vi "Begin.vi"() -> (0 "error out":errorcluster)   [LabVIEW 2013]
doc: "Called before other user functions, this VI is expected to open initial I/O refnums, load in file data, and do all program initialization. Notice that the <B>error out</B> terminal is simply used for data flow. Wiring it to other structures or subVIs ensures that this VI runs first."
uses:
  <vilib>/Rock Robotics/WPI/Joystick/WPI_JoystickDeviceEnum.ctl
  <vilib>/Rock Robotics/SystemInterfaces/Typedef/FPGA_TypedefDigitalModule.ctl
  <vilib>/Rock Robotics/SystemInterfaces/DIO/FPGA_DIOChannel.ctl
  <vilib>/Rock Robotics/SystemInterfaces/DIO/FPGA_DIORelayChannel.ctl
  <vilib>/Rock Robotics/SystemInterfaces/Typedef/FPGA_TypedefSolenoidModule.ctl
  <vilib>/Rock Robotics/WPI/Solenoid/WPI_SolenoidChannel.ctl
  <vilib>/Rock Robotics/WPI/Solenoid/WPI_SolenoidValue.ctl
  <vilib>/Rock Robotics/SystemInterfaces/DIO/FPGA_DIOPWMChannel.ctl
  <vilib>/Rock Robotics/WPI/Solenoid/WPI_SolenoidOpenDouble.vi
  <vilib>/Rock Robotics/WPI/Solenoid/WPI_SolenoidSetEnum.vi
  <vilib>/Rock Robotics/WPI/Counter/WPI_CounterDigitalInputToDigitalSource.vi
  <vilib>/Rock Robotics/WPI/RobotDrive/WPI_RobotDriveOpen2MotorWithVictor.vi
  <vilib>/Rock Robotics/WPI/Compressor/WPI_CompressorGetSetRefNum.vi
  <vilib>/Rock Robotics/WPI/Camera/WPI_CameraImageSize.ctl
  <vilib>/Rock Robotics/WPI/Camera/WPI_CameraWhite Balance Values.ctl
  <vilib>/Rock Robotics/WPI/Camera/WPI_CameraExposure Values.ctl
  <vilib>/Rock Robotics/WPI/Camera/WPI_CameraFrameRate.ctl
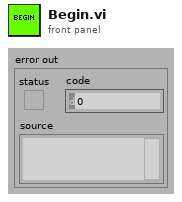
[diagram p1: front panel]
types:
  T1 = typedef "FPGA_DIOChannel.ctl" = enum8{"DIO 1", "DIO 2", "DIO 3", "DIO 4", "DIO 5", "DIO 6", "DIO 7", "DIO 8", "DIO 9", "DIO 10", "DIO 11", "DIO 12", "DIO 13", "DIO 14", "Invalid"}
  T2 = typedef "FPGA_DIOPWMChannel.ctl" = enum8{"PWM 1", "PWM 2", "PWM 3", "PWM 4", "PWM 5", "PWM 6", "PWM 7", "PWM 8", "PWM 9", "PWM 10", "Invalid"}
  T3 = typedef "WPI_SolenoidValue.ctl" = enum16{"Off", "On", "Forward", "Reverse"}
  T4 = typedef "WPI_SolenoidChannel.ctl" = enum8{"Solenoid 1", "Solenoid 2", "Solenoid 3", "Solenoid 4", "Solenoid 5", "Solenoid 6", "Solenoid 7", "Solenoid 8", "Invalid"}
  T5 = typedef "FPGA_TypedefSolenoidModule.ctl" = enum16{"Solenoid Module 1", "Solenoid Module 2"}
  T6 = typedef "FPGA_DIORelayChannel.ctl" = enum8{"Relay 1", "Relay 2", "Relay 3", "Relay 4", "Relay 5", "Relay 6", "Relay 7", "Relay 8", "Invalid"}
  T7 = typedef "WPI_JoystickDeviceEnum.ctl" = enum16{"USB 1", "USB 2", "USB 3", "USB 4", "Kinect 1", "Kinect 2"}
  T8 = typedef "FPGA_TypedefDigitalModule.ctl" = enum16{"Digital Module 1", "Digital Module 2"}
  T9 = typedef "WPI_CameraFrameRate.ctl" = u32
  T10 = typedef "WPI_CameraExposure Values.ctl" = enum16{"Auto", "Flicker-free 50 Hz", "Flicker-free 60 Hz", "Hold current"}
  T11 = typedef "WPI_CameraWhite Balance Values.ctl" = enum16{"Auto", "Fixed indoor", "Fixed outdoor 1", "Fixed outdoor 2", "Fixed fluorescent 1", "Fixed fluorescent 2", "Hold current"}
  T12 = typedef "WPI_CameraImageSize.ctl" = enum16{"640x480", "320x240", "160x120"}
  T13 = typedef "WPI_CameraDevRef.ctl" = cluster{"Camera Address":string, "CameraStatus":errorcluster, "Acquire Image Notifier":refnum<notifier>}
  T14 = typedef "WPI_SolenoidDevRef.ctl" = cluster{"DevStatus":errorcluster, "Solenoid Module":T5, "Forward Solenoid Channel":T4, "Reverse Solenoid Channel":T4}
  T15 = typedef "WPI_DigitalInputDevRef.ctl" = cluster{"DevStatus":errorcluster, "DIO Channel":T1, "Digital Module":T8}
  T16 = typedef "WPI_RobotDriveDevRef.ctl" = cluster{"DevStatus":errorcluster, "Motors[]":T17[], "Square Inputs":bool, "Max Output":dbl, "Isochronous":bool}
  T17 = typedef "WPI_MotorControlDeviceRef.ctl" = cluster{"DeviceStatus":errorcluster, "Type":enum16{"PWM", "CAN"}, "PWM":cluster{"Digital Module":T8, "PWM Channel":T2, "DeadBand":T18}, "CAN":cluster{"Device Number":u8, "Control Mode":T19, "Semaphore":T20, "Max Vout":dbl}, "Invert":bool, "TransformRef":T21, "InvTransformRef":T21}
  T18 = typedef "WPI_PWMDeadband.ctl" = cluster{"Name":string, "maxPositivePwm":i32, "minPositivePwm":i32, "centerPwm":i32, "maxNegativePwm":i32, "minNegativePwm":i32, "angularRange":u16}
  T19 = typedef "WPI_CANJaguar_ControlMode.ctl" = enum8{"Percent VBus", "Current", "Speed", "Position", "Voltage"}
  T20 = typedef "Semaphore RefNum" = refnum<k1>
  T21 = typedef "WPI_PWMTransform_ConPane.ctl" = refnum<vi>
  T22 = typedef "WPI_CompressorDevRef.ctl" = cluster{"DevStatus":errorcluster, "DigitalInputDevRef":T15, "RelayDevRef":T23}
  T23 = typedef "WPI_RelayDevRef.ctl" = cluster{"DevStatus":errorcluster, "Relay Channel":T6, "Digital Module":T8, "Relay Direction":T24}
  T24 = typedef "WPI_RelayDirection.ctl" = enum16{"Both directions", "Forward only", "Reverse only"}
  T25 = typedef "FPGA_CounterEncoderSourceConvertionLVSourceType.ctl" = cluster{"DevStatus":errorcluster, "AnalogTriggerMode?":bool, "DigitalMode":cluster{"Digital Module":T8, "DIO Channel":T26}, "AnalogTriggerMode":cluster{"AnalogTriggerIndex":T27, "OutputType":T28}}
  T26 = typedef "FPGA_DIODigitalSourceChannel.ctl" = enum8{"DIO 1", "DIO 2", "DIO 3", "DIO 4", "DIO 5", "DIO 6", "DIO 7", "DIO 8", "DIO 9", "DIO 10", "DIO 11", "DIO 12", "DIO 13", "DIO 14", "Disabled"}
  T27 = typedef "FPGA_AnalogTriggerIndex.ctl" = enum8{"Trig 0", "Trig 1", "Trig 2", "Trig 3", "Trig 4", "Trig 5", "Trig 6", "Trig 7", "Invalid"}
  T28 = typedef "FPGA_AnalogTriggerOutType.ctl" = enum16{"InWindow", "TriggerState", "Rising", "Falling"}
  T29 = typedef "WPI_EncoderDevRef.ctl" = cluster{"DevStatus":errorcluster, "EncoderIndex":T30, "CounterIndex":T31, "DistancePerCount":dbl, "Decoding Type":T32}
  T30 = typedef "FPGA_EncoderIdx.ctl" = enum8{"Enc 0", "Enc 1", "Enc 2", "Enc 3", "Invalid"}
  T31 = typedef "FPGA_CounterCtrSystemIndex.ctl" = enum8{"Ctr 0", "Ctr 1", "Ctr 2", "Ctr 3", "Ctr 4", "Ctr 5", "Ctr 6", "Ctr 7", "Invalid"}
  T32 = typedef "WPI_EncoderType.ctl" = enum16{"1x", "2x", "4x"}
  T33 = typedef "WPI_JoystickDevRef.ctl" = cluster{"Device":T7}
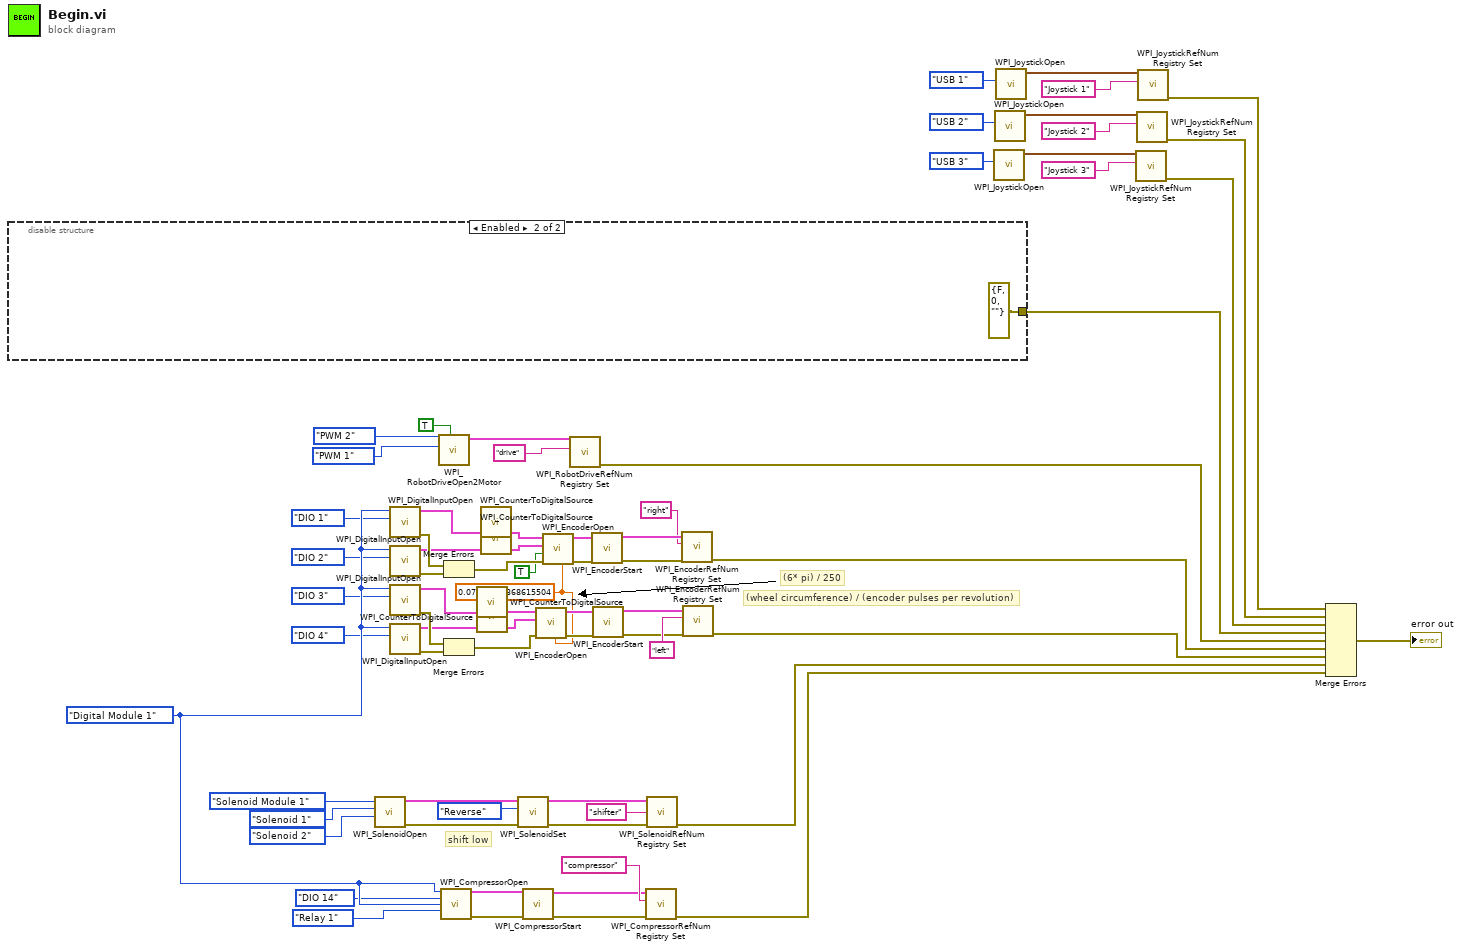
[diagram p0: block diagram]
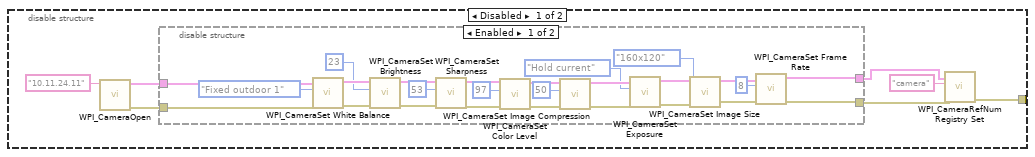
[diagram p2: hidden frame]
diagram:
  w11 = 0.07539822368615504 ("DistancePerCount")
  w54 = FPGA_TypedefDigitalModule."Digital Module 1" ("Digital Module (Module 1)")
  # "shift low"
  # "(wheel circumference) / (encoder pulses per revolution)"
  # "(6* pi) / 250"
  n1 = disable-structure shown="Enabled" {
    disable-tunnel: [w72 errorcluster {"status"=FALSE, "code"=0, "source"=""} ("error out")] -> w59
    frame Disabled {
      n2 = call <vilib>:"WPI_CameraOpen.vi"("Camera Address"="10.11.24.11") -> ("error out"=w74:errorcluster, "CameraDevRef"=w76:T13)  [unwired: 9 in]
      n3 = disable-structure shown="Enabled" {
        disable-tunnel: w76 -> [w102 w106]
        disable-tunnel: [w80 w106] -> w75
        disable-tunnel: w74 -> [w89 w105]
        disable-tunnel: [w79 w105] -> w73
        frame Enabled {
          n4 = call <vilib>:"WPI_CameraSet White Balance.vi"("error in (no error)"=w89, "White Balance"=WPI_CameraWhite_Balance_Values."Fixed outdoor 1", "CameraDevRef"=w102) -> ("error out"=w90:errorcluster, "CameraDevRef Out"=w101:T13)  [unwired: 7 in]
          n5 = call <vilib>:"WPI_CameraSet Brightness.vi"("error in (no error)"=w90, "Brightness"=23, "CameraDevRef"=w101) -> ("error out"=w91:errorcluster, "CameraDevRef Out"=w100:T13)  [unwired: 7 in]
          n6 = call <vilib>:"WPI_CameraSet Sharpness.vi"("error in (no error)"=w91, "Sharpness"=53, "CameraDevRef"=w100) -> ("error out"=w92:errorcluster, "CameraDevRef Out"=w99:T13)  [unwired: 7 in]
          n7 = call <vilib>:"WPI_CameraSet Color Level.vi"("error in (no error)"=w92, "Color Level"=97, "CameraDevRef"=w99) -> ("error out"=w93:errorcluster, "CameraDevRef Out"=w98:T13)  [unwired: 7 in]
          n8 = call <vilib>:"WPI_CameraSet Image Compression.vi"("error in (no error)"=w93, "Compression"=50, "CameraDevRef"=w98) -> ("error out"=w104:errorcluster, "CameraDevRef Out"=w103:T13)  [unwired: 7 in]
          n9 = call <vilib>:"WPI_CameraSet Exposure.vi"("error in (no error)"=w104, "Exposure"=WPI_CameraExposure_Values."Hold current", "CameraDevRef"=w103) -> ("error out"=w94:errorcluster, "CameraDevRef Out"=w97:T13)  [unwired: 7 in]
          n10 = call <vilib>:"WPI_CameraSet Image Size.vi"("error in (no error)"=w94, "Image Size"=WPI_CameraImageSize."160x120", "CameraDevRef"=w97) -> ("error out"=w95:errorcluster, "CameraDevRef Out"=w96:T13)  [unwired: 7 in]
          n11 = call <vilib>:"WPI_CameraSet Frame Rate.vi"("error in (no error)"=w95, "Frame Rate (fps)"=T9 8, "CameraDevRef"=w96) -> ("error out"=w79:errorcluster, "CameraDevRef Out"=w80:T13)  [unwired: 7 in]
        }
        frame Disabled {
        }
      }
      n12 = call <vilib>:"WPI_CameraRefNum Registry Set.vi"("error in (no error)"=w73, "refnum name"="camera", "CameraDevRef"=w75) -> ("error out"=w72:errorcluster)  [unwired: 7 in, 1 out]
    }
    frame Enabled {
    }
  }
  n13 = call-poly <vilib>:"WPI_SolenoidOpen.vi"("Reverse Solenoid Channel"=WPI_SolenoidChannel."Solenoid 2", "Forward Solenoid Channel"=WPI_SolenoidChannel."Solenoid 1", "Solenoid Module (Module 1)"=FPGA_TypedefSolenoidModule."Solenoid Module 1") -> ("error out"=w38:errorcluster, "SolenoidDevRef"=w39:T14)  [unwired: 7 in]
  n14 = call <vilib>:"WPI_DigitalInputOpen.vi"("DIO Channel"=FPGA_DIOChannel."DIO 1", "Digital Module (Module 1)"=w54) -> ("error out"=w5:errorcluster, "DigitalInputDevRef"=w19:T15)  [unwired: 8 in]
  n15 = call <vilib>:"WPI_DigitalInputOpen.vi"("DIO Channel"=FPGA_DIOChannel."DIO 2", "Digital Module (Module 1)"=w54) -> ("error out"=w7:errorcluster, "DigitalInputDevRef"=w4:T15)  [unwired: 8 in]
  n16 = call <vilib>:"WPI_DigitalInputOpen.vi"("DIO Channel"=FPGA_DIOChannel."DIO 3", "Digital Module (Module 1)"=w54) -> ("error out"=w8:errorcluster, "DigitalInputDevRef"=w33:T15)  [unwired: 8 in]
  n17 = call <vilib>:"WPI_DigitalInputOpen.vi"("DIO Channel"=FPGA_DIOChannel."DIO 4", "Digital Module (Module 1)"=w54) -> ("error out"=w10:errorcluster, "DigitalInputDevRef"=w3:T15)  [unwired: 8 in]
  n18 = call-poly <vilib>:"WPI_RobotDriveOpen2Motor.vi"("Left Motor Inverted"=TRUE, "Right Motor"=FPGA_DIOPWMChannel."PWM 1", "Left Motor"=FPGA_DIOPWMChannel."PWM 2") -> ("RobotDriveDevRef"=w35:T16)  [unwired: 7 in, 1 out]
  n19 = call <vilib>:"WPI_CompressorOpen.vi"("Pressure Switch Digital Module (Module 1)"=w54, "Pressure Switch DIO Channel"=FPGA_DIOChannel."DIO 14", "Relay Digital Module (Module 1)"=w54, "Relay Channel"=FPGA_DIORelayChannel."Relay 1") -> ("CompressorDevRef"=w48:T22, "error out"=w47:errorcluster)  [unwired: 10 in]
  n20 = Merge Errors(w5, w7) -> (w6:errorcluster)
  n21 = Merge Errors(w8, w10) -> (w9:errorcluster)
  n22 = call-poly <vilib>:"WPI_CounterToDigitalSource.vi"("DigitalInputDevRef"=w33) -> ("Digital Source"=w26:T25)  [unwired: 6 in]
  n23 = call-poly <vilib>:"WPI_CounterToDigitalSource.vi"("DigitalInputDevRef"=w3) -> ("Digital Source"=w27:T25)  [unwired: 6 in]
  n24 = call-poly <vilib>:"WPI_CounterToDigitalSource.vi"("DigitalInputDevRef"=w19) -> ("Digital Source"=w25:T25)  [unwired: 6 in]
  n25 = call-poly <vilib>:"WPI_CounterToDigitalSource.vi"("DigitalInputDevRef"=w4) -> ("Digital Source"=w24:T25)  [unwired: 6 in]
  n26 = call-poly <vilib>:"WPI_SolenoidSet.vi"("error in (no error)"=w38, "Value"=WPI_SolenoidValue."Reverse", "SolenoidDevRef"=w39) -> ("error out"=w37:errorcluster, "SolenoidDevRef"=w36:T14)  [unwired: 7 in]
  n27 = call <vilib>:"WPI_CompressorStart.vi"("error in (no error)"=w47, "CompressorDevRef"=w48) -> ("error out"=w46:errorcluster, "CompressorDevRef"=w45:T22)  [unwired: 8 in]
  n28 = call <vilib>:"WPI_EncoderOpen.vi"("DistancePerCount"=w11, "error in (no error)"=w9, "BSource"=w27, "ASource"=w26) -> ("error out"=w28:errorcluster, "EncoderDevRef"=w29:T29)  [unwired: 6 in]
  n29 = call <vilib>:"WPI_EncoderOpen.vi"("DistancePerCount"=w11, "error in (no error)"=w6, "Invert Direction (False)"=TRUE, "BSource"=w24, "ASource"=w25) -> ("error out"=w23:errorcluster, "EncoderDevRef"=w22:T29)  [unwired: 5 in]
  n30 = call <vilib>:"WPI_RobotDriveRefNum Registry Set.vi"("refnum name"="drive", "RobotDriveDevRef"=w35) -> ("error out"=w58:errorcluster)  [unwired: 8 in, 1 out]
  n31 = call <vilib>:"WPI_EncoderStart.vi"("error in (no error)"=w23, "EncoderDevRef"=w22) -> ("error out"=w21:errorcluster, "EncoderDevRef"=w20:T29)  [unwired: 8 in]
  n32 = call <vilib>:"WPI_EncoderStart.vi"("error in (no error)"=w28, "EncoderDevRef"=w29) -> ("error out"=w30:errorcluster, "EncoderDevRef"=w31:T29)  [unwired: 8 in]
  n33 = call <vilib>:"WPI_CompressorRefNum Registry Set.vi"("error in (no error)"=w46, "refnum name"="compressor", "CompressorDevRef"=w45) -> ("error out"=w52:errorcluster)  [unwired: 7 in, 1 out]
  n34 = call <vilib>:"WPI_SolenoidRefNum Registry Set.vi"("error in (no error)"=w37, "refnum name"="shifter", "SolenoidDevRef"=w36) -> ("error out"=w53:errorcluster)  [unwired: 7 in, 1 out]
  n35 = call <vilib>:"WPI_EncoderRefNum Registry Set.vi"("error in (no error)"=w21, "refnum name"="right", "EncoderDevRef"=w20) -> ("error out"=w57:errorcluster)  [unwired: 7 in, 1 out]
  n36 = call <vilib>:"WPI_EncoderRefNum Registry Set.vi"("error in (no error)"=w30, "refnum name"="left", "EncoderDevRef"=w31) -> ("error out"=w56:errorcluster)  [unwired: 7 in, 1 out]
  n37 = call <vilib>:"WPI_JoystickOpen.vi"("JoystickDevice"=WPI_JoystickDeviceEnum."USB 3") -> ("JoystickDevRef"=w70:T33)  [unwired: 10 in]
  n38 = call <vilib>:"WPI_JoystickOpen.vi"("JoystickDevice"=WPI_JoystickDeviceEnum."USB 2") -> ("JoystickDevRef"=w67:T33)  [unwired: 10 in]
  n39 = call <vilib>:"WPI_JoystickOpen.vi"("JoystickDevice"=WPI_JoystickDeviceEnum."USB 1") -> ("JoystickDevRef"=w64:T33)  [unwired: 10 in]
  n40 = call <vilib>:"WPI_JoystickRefNum Registry Set.vi"("refnum name"="Joystick 3", "JoystickDevRef"=w70) -> ("error out"=w60:errorcluster)  [unwired: 8 in, 1 out]
  n41 = call <vilib>:"WPI_JoystickRefNum Registry Set.vi"("refnum name"="Joystick 2", "JoystickDevRef"=w67) -> ("error out"=w61:errorcluster)  [unwired: 8 in, 1 out]
  n42 = call <vilib>:"WPI_JoystickRefNum Registry Set.vi"("refnum name"="Joystick 1", "JoystickDevRef"=w64) -> ("error out"=w62:errorcluster)  [unwired: 8 in, 1 out]
  n43 = Merge Errors(w62, w61, w60, w59, w58, w57, w56, w53, w52) -> (→"error out":errorcluster)
